vi "Constructor.vi"(8 "error in":errorcluster, 11 "Baseline Mocon \npiD-Tech plus in":refnum<class "Baseline Mocon piD-Tech plus.lvclass">) -> (0 "error out":errorcluster, 2 "init":bool, 3 "Baseline Mocon \npiD-Tech plus out":refnum<class "Baseline Mocon piD-Tech plus.lvclass">)   [LabVIEW 2011, in "Baseline Mocon piD-Tech plus.lvclass"]
uses:
  Baseline Mocon piD-Tech plus.lvclass
  Baseline Mocon piD-Tech plus.lvclass/Baseline Mocon piD-Tech plus.ctl
  <vilib>/DAQmx/create/channels.llb/DAQmx Create Channel (AI-Voltage-Basic).vi
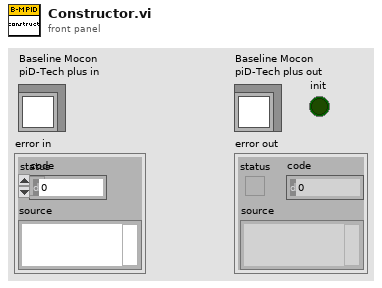
[diagram p1: front panel]
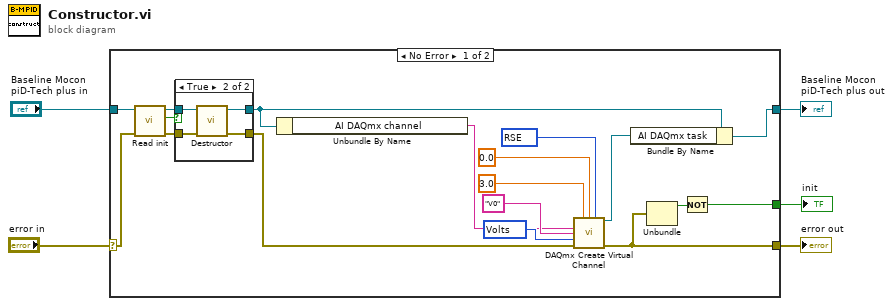
[diagram p0: block diagram]
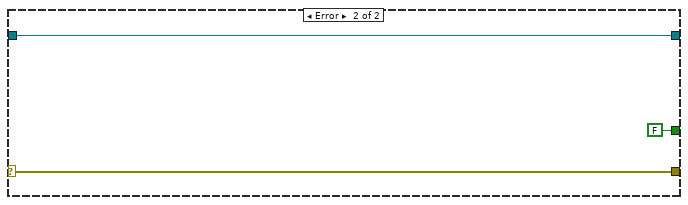
[diagram p3: hidden frame]
diagram:
  n1 = case shown="No Error" "error in" {
    selector: "error in" -> [w19 w32]
    tunnel: [w9 w32] -> w4
    tunnel: [w6 w31] -> w2
    tunnel: "Baseline Mocon \npiD-Tech plus in" -> [w20 w31]
    tunnel: [w7 FALSE] -> w1
    frame No Error {
      w18 = 10083 items=["default"=-1, "RSE"=10083, "NRSE"=10078, "Differential"=10106, "Pseudodifferential"=12529] ("input terminal configuration")
      w15 = 10348 items=["Volts"=10348, "From Custom Scale"=10065] ("V0 units")
      n2 = call-dynamic "Read init.vi"("error in (no error)"=w19, "Detector in"=w20) -> ("error out"=w22:errorcluster, "init"=w21:bool, "Detector out"=w23:refnum<class "Baseline Mocon piD-Tech plus.lvclass">)  [unwired: 7 in]
      n3 = case shown="True" w21 {
        tunnel: w22 -> [w24 w28]
        tunnel: w23 -> [w25 w29]
        tunnel: [w25 w27] -> w11
        tunnel: [w24 w26] -> w12
        frame False {
        }
        frame True {
          n4 = call-dynamic "Destructor.vi"("error in"=w28, "Baseline Mocon \npiD-Tech plus in"=w29) -> ("error out"=w26:errorcluster, "Baseline Mocon \npiD-Tech plus out"=w27:refnum<class "Baseline Mocon piD-Tech plus.lvclass">)  [unwired: 8 in]
        }
      }
      n5 = Unbundle By Name(w11) -> ("AI DAQmx channel"=w13:tag)
      n6 = call-poly <vilib>:"DAQmx Create Virtual Channel.vi"("maximum value"=3.0, "minimum value"=0.0, "input terminal configuration"=w18, "physical channels"=w13, "name to assign"="V0", "units"=w15, "error in"=w12) -> ("task out"=w10:refnum<k21>, "error out"=w9:errorcluster)  [unwired: 7 in]
      n7 = Bundle By Name(cluster=w11, "AI DAQmx task"=w10) -> (w6:refnum<class "Baseline Mocon piD-Tech plus.lvclass">)
      n8 = Unbundle(w9) -> ("status"=w8:bool)  [unwired: 2 out]
      n9 = Not(x=w8) -> (.not. x?=w7:bool)
    }
    frame Error {
    }
  }
  "error out" <- w4
  "Baseline Mocon \npiD-Tech plus out" <- w2
  "init" <- w1
